vi "GetTagValue_U64.vi"(6 "error in (no error)":errorcluster caption="Fehler (Eingang, kein Fehler)", 7 "Tag Code":u16, 8 "Directory Entries":T2[](array[typedef]) {"Value" format="%.0x"}, 9 "TIFF file":T1 {"BigTiff,Endian" items=["Big-Endian"=0, "Native"=1, "Little-Endian"=2, "BigTiff-Big-Endian"=256, "Bigtiff,Native"=257, "Biftiff,Littleendian"=258]}) -> (0 "error out":errorcluster caption="Fehler (Ausgang)", 1 "Index (not found = -1)":i32, 2 "Single Value":u64, 3 "TIFF file out":T1 {"BigTiff,Endian" items=["Big-Endian"=0, "Native"=1, "Little-Endian"=2, "BigTiff-Big-Endian"=256, "Bigtiff,Native"=257, "Biftiff,Littleendian"=258]})   [LabVIEW 2011]
uses:
  IFD.ctl
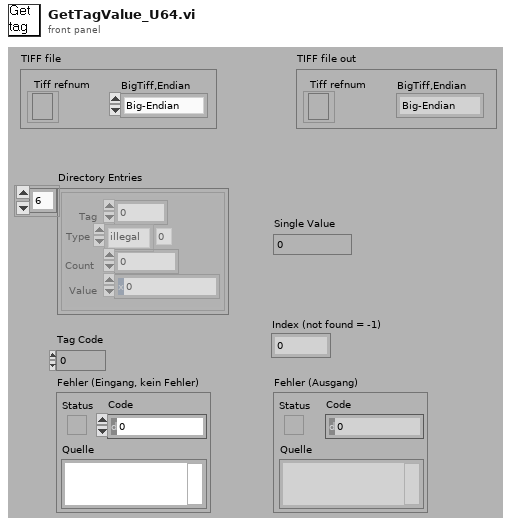
[diagram p1: front panel]
types:
  T1 = cluster{"Tiff refnum":refnum<file>, "BigTiff,Endian":u16}
  T2 = typedef "IFD.ctl" = cluster{"Tag":u16, "Type":enum16{"illegal", "Byte", "Ascii", "Short", "Long", "Rational", "SByte", "Undefined", "SShort", "SLong", "SRational 2xSLong", "Float 4byte", "Double 8Byte", "No13", "No14", "No15", "U64", "I64", "U64-IFD8"}, "Count":u64, "Value":u64}
  T3 = enum16{"illegal", "Byte", "Ascii", "Short", "Long", "Rational", "SByte", "Undefined", "SShort", "SLong", "SRational 2xSLong", "Float 4byte", "Double 8Byte", "No13", "No14", "No15", "U64", "I64", "U64-IFD8"}[]
  T4 = enum16{"illegal", "Byte", "Ascii", "Short", "Long", "Rational", "SByte", "Undefined", "SShort", "SLong", "SRational 2xSLong", "Float 4byte", "Double 8Byte", "No13", "No14", "No15", "U64", "I64", "U64-IFD8"}
  T5 = cluster{"byte stream type":u32, "byte stream type 2":u32}
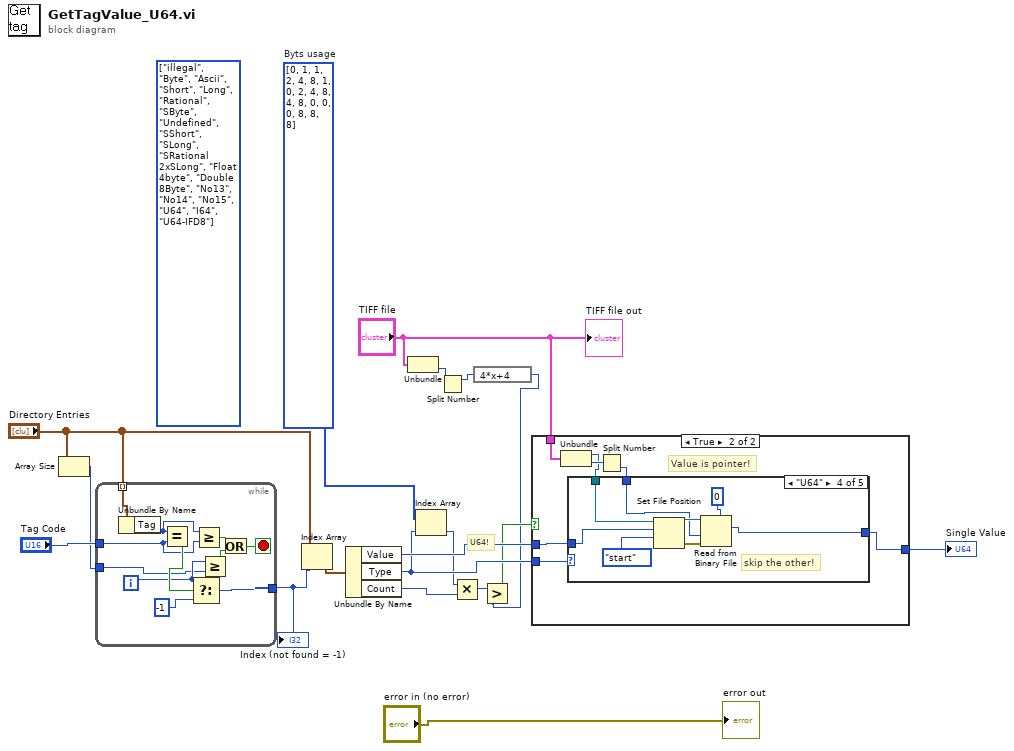
[diagram p0: block diagram]
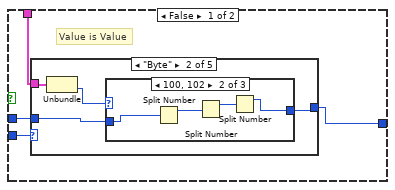
[diagram p2: hidden frame]
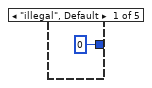
[diagram p3: hidden frame]
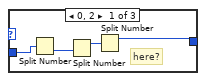
[diagram p4: hidden frame]
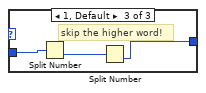
[diagram p5: hidden frame]
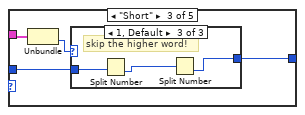
[diagram p6: hidden frame]
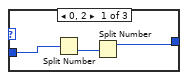
[diagram p7: hidden frame]
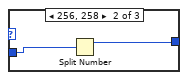
[diagram p8: hidden frame]
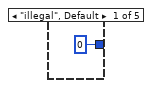
[diagram p11: hidden frame]
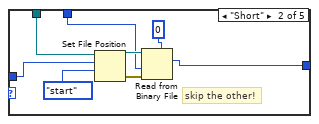
[diagram p12: hidden frame]
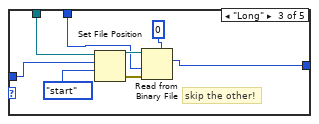
[diagram p13: hidden frame]
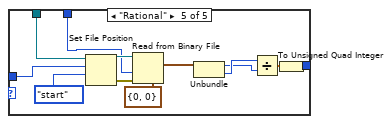
[diagram p14: hidden frame]
diagram:
  w11 = i32[] [0, 1, 1, 2, 4, 8, 1, 0, 2, 4, 8, 4, 8, 0, 0, 0, 8, 8, 8]  # Byts usage
  (unwired) T3 [enum."illegal", enum."Byte", enum."Ascii", enum."Short", enum."Long", enum."Rational", enum."SByte", enum."Undefined", enum."SShort", enum."SLong", enum."SRational 2xSLong", enum."Float 4byte", enum."Double 8Byte", enum."No13", enum."No14", enum."No15", enum."U64", enum."I64", enum."U64-IFD8"] items=["illegal", "Byte", "Ascii", "Short", "Long", "Rational", "SByte", "Undefined", "SShort", "SLong", "SRational 2xSLong", "Float 4byte", "Double 8Byte", "No13", "No14", "No15", "U64", "I64", "U64-IFD8"]
  # "U64!"
  n1 = Array Size(array="Directory Entries") -> (size(s)=w13:i32)
  n2 = while {
    tunnel: "Directory Entries" -> [w29] mode=indexing
    tunnel: "Tag Code" -> [w26]
    tunnel: [w24] -> w15
    tunnel: w13 -> [w22]
    i -> [w23]
    stop <- w21 stop-if-true
    n3 = Unbundle By Name(w29) -> ("Tag"=w27:u16)
    n4 = Equal?(x=w27, y=w26) -> (x = y?=w28:bool)
    n5 = Select(t=w23, s=w28, f=-1) -> (s? t:f=w24:i32)
    n6 = Greater Or Equal?(x=w27, y=w26) -> (x >= y?=w20:bool)
    n7 = Greater Or Equal?(x=w23, y=w22) -> (x >= y?=w19:bool)
    n8 = Or(x=w20, y=w19) -> (x .or. y?=w21:bool)
  }
  "Index (not found = -1)" <- w15
  n9 = Index Array(array="Directory Entries", index=w15) -> (element=w17:T2)
  n10 = Unbundle By Name(w17) -> ("Value"=w16:u64, "Type"=w12:T4, "Count"=w9:u64)
  n11 = Unbundle("TIFF file") -> ("BigTiff,Endian"=w5:u16)  [unwired: 1 out]
  n12 = Index Array(array=w11, index=w12) -> (element=w10:i32)
  n13 = Split Number(x=w5) -> (hi(x)=w4:u8)  [unwired: 1 out]
  n14 = Multiply(x=w10, y=w9) -> (x*y=w8:u64)
  n15 = expression code="4*x+4"(w4) -> (w2:u8)
  n16 = Greater?(x=w8, y=w2) -> (0:w6:bool)
  n17 = case shown="True" w6 {
    tunnel: w16 -> [w33 w70]
    tunnel: "TIFF file" -> [w32 w67]
    tunnel: w12 -> [w31 w69]
    tunnel: [w30 w68] -> w7
    frame False {
      # "Value is Value"
      n18 = case shown="\"Byte\"" w31 {
        tunnel: w32 -> [_ w38 w51 _ _]
        tunnel: w33 -> [_ w36 w53 w62 w63]
        tunnel: [u32 0 ("Value") w35 w52 w62 w63] -> w30
        frame "illegal", Default {
        }
        frame "Byte" {
          n19 = Unbundle(w38) -> ("BigTiff,Endian"=w37:u16)  [unwired: 1 out]
          n20 = case shown="100, 102" w37 {
            tunnel: w36 -> [w40 w45 w49]
            tunnel: [w41 w43 w47] -> w35
            frame 0, 2 {
              # "here?"
              n21 = Split Number(x=w40) -> (lo(x)=w39:u32)  [unwired: 1 out]
              n22 = Split Number(x=w39) -> (hi(x)=w42:u16)  [unwired: 1 out]
              n23 = Split Number(x=w42) -> (hi(x)=w41:u8)  [unwired: 1 out]
            }
            frame 256, 258 {
              n24 = Split Number(x=w45) -> (hi(x)=w46:u32)  [unwired: 1 out]
              n25 = Split Number(x=w46) -> (hi(x)=w44:u16)  [unwired: 1 out]
              n26 = Split Number(x=w44) -> (hi(x)=w43:u8)  [unwired: 1 out]
            }
            frame 1, Default {
              # "skip the higher word!"
              n27 = Split Number(x=w49) -> (lo(x)=w48:u32)  [unwired: 1 out]
              n28 = Split Number(x=w48) -> (lo(x)=w47:u16)  [unwired: 1 out]
            }
          }
        }
        frame "Short" {
          n29 = Unbundle(w51) -> ("BigTiff,Endian"=w50:u16)  [unwired: 1 out]
          n30 = case shown="1, Default" w50 {
            tunnel: w53 -> [w55 w58 w60]
            tunnel: [w56 w57 w61] -> w52
            frame 0, 2 {
              n31 = Split Number(x=w55) -> (lo(x)=w54:u32)  [unwired: 1 out]
              n32 = Split Number(x=w54) -> (hi(x)=w56:u16)  [unwired: 1 out]
            }
            frame 256, 258 {
              n33 = Split Number(x=w58) -> (hi(x)=w57:u32)  [unwired: 1 out]
            }
            frame 1, Default {
              # "skip the higher word!"
              n34 = Split Number(x=w60) -> (lo(x)=w59:u32)  [unwired: 1 out]
              n35 = Split Number(x=w59) -> (lo(x)=w61:u16)  [unwired: 1 out]
            }
          }
        }
        frame "Long" {
        }
        frame "U64", "I64" {
        }
      }
    }
    frame True {
      # "Value is pointer!"
      n36 = Unbundle(w67) -> ("Tiff refnum"=w64:refnum<file>, "BigTiff,Endian"=w66:u16)
      n37 = Split Number(x=w66) -> (lo(x)=w65:u8)  [unwired: 1 out]
      n38 = case shown="\"U64\"" w69 {
        tunnel: w70 -> [_ w75 w84 w92 w106]
        tunnel: [u32 0 ("Value") w74 w82 w90 w100] -> w68
        tunnel: w65 -> [_ w72 w80 w88 w98]
        tunnel: w64 -> [_ w73 w81 w89 w99]
        frame "illegal", Default {
        }
        frame "Short" {
          # "skip the other!"
          n39 = Set File Position(offset (in bytes) (0)=w75, refnum=w73, from (0:start)=enum16{"start", "end", "current"}."start" ("pos mode (0:2)")) -> (refnum out=w78:refnum<file>, error out=w77:errorcluster)  [unwired: 1 in]
          n40 = Read from Binary File(5:u32 0 ("byte stream type"), 8:w77, 9:w72, 11:w78) -> (2:w74:u32)  [unwired: 5 out]
        }
        frame "Long" {
          # "skip the other!"
          n41 = Set File Position(offset (in bytes) (0)=w84, refnum=w81, from (0:start)=enum16{"start", "end", "current"}."start" ("pos mode (0:2)")) -> (refnum out=w86:refnum<file>, error out=w85:errorcluster)  [unwired: 1 in]
          n42 = Read from Binary File(5:u32 0 ("byte stream type"), 8:w85, 9:w80, 11:w86) -> (2:w82:u32)  [unwired: 5 out]
        }
        frame "U64" {
          # "skip the other!"
          n43 = Set File Position(offset (in bytes) (0)=w92, refnum=w89, from (0:start)=enum16{"start", "end", "current"}."start" ("pos mode (0:2)")) -> (refnum out=w94:refnum<file>, error out=w93:errorcluster)  [unwired: 1 in]
          n44 = Read from Binary File(5:u64 0 ("byte stream type"), 8:w93, 9:w88, 11:w94) -> (2:w90:u64)  [unwired: 5 out]
        }
        frame "Rational" {
          n45 = Set File Position(offset (in bytes) (0)=w106, refnum=w99, from (0:start)=enum16{"start", "end", "current"}."start" ("pos mode (0:2)")) -> (refnum out=w103:refnum<file>, error out=w102:errorcluster)  [unwired: 1 in]
          n46 = Read from Binary File(5:T5 {"byte stream type"=0, "byte stream type 2"=0}, 8:w102, 9:w98, 11:w103) -> (2:w101:T5)  [unwired: 5 out]
          n47 = Unbundle(w101) -> ("byte stream type"=w96:u32, "byte stream type 2"=w97:u32)
          n48 = Divide(x=w97, y=w96) -> (x/y=w104:dbl)
          n49 = To Unsigned Quad Integer(1:w104) -> (0:w100:u64)
        }
      }
    }
  }
  "Single Value" <- w7
  "error out" <- "error in (no error)"
  "TIFF file out" <- "TIFF file"
